vi "Write Required Relative Epsilon.vi"(10 "Required Relative Epsilon":dbl=6.0, 11 "Floating Point in":refnum<class "Floating Point.lvclass">) -> (3 "Floating Point out":refnum<class "Floating Point.lvclass">)   [LabVIEW 2018, in "Floating Point.lvclass"]
uses:
  Floating Point.lvclass
  Floating Point.lvclass/Floating Point.ctl
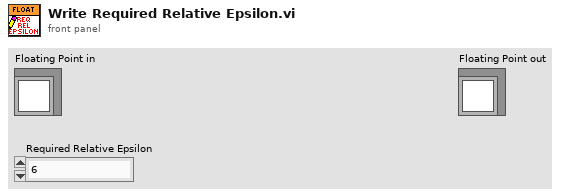
[diagram p1: front panel]
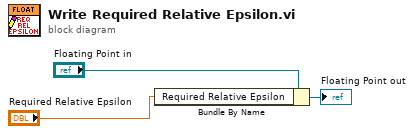
[diagram p0: block diagram]
diagram:
  n1 = Bundle By Name(cluster="Floating Point in", "Required Relative Epsilon"="Required Relative Epsilon") -> (→"Floating Point out":refnum<class "Floating Point.lvclass">)
